vi "SetStyle.vi"(8 "error in (no error)":errorcluster, 10 "Style":T1(ring), 11 "Pen in":refnum<class "Pen.lvclass">) -> (0 "error out":errorcluster, 3 "Pen out":refnum<class "Pen.lvclass">)   [LabVIEW 2021, in "Picture2D.lvlib" / "Pen.lvclass"]
uses:
  Pen.lvclass
  Pen.lvclass/Pen.ctl
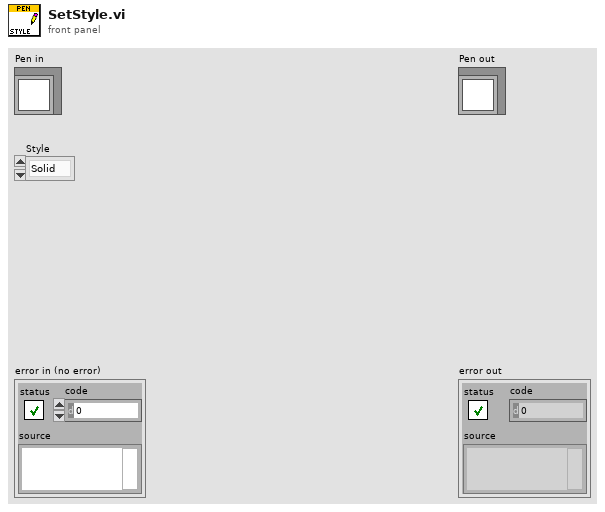
[diagram p1: front panel]
types:
  T1 = enum32{"Solid", "Dash", "Dot", "DashDot", "DashDotDot"}
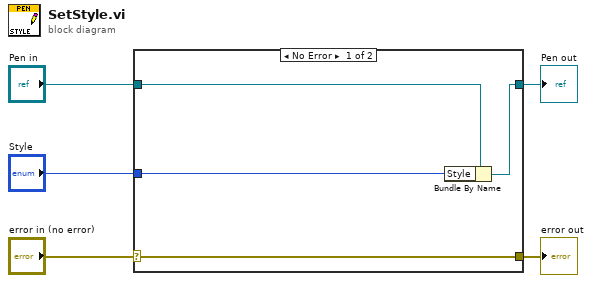
[diagram p0: block diagram]
diagram:
  n1 = case shown="No Error" "error in (no error)" {
    selector: "error in (no error)" -> [w9 w10]
    tunnel: [w9 w10] -> w4
    tunnel: [w7 w11] -> w2
    tunnel: "Pen in" -> [w8 w11]
    tunnel: "Style" -> [w6 _]
    frame No Error {
      n2 = Bundle By Name(cluster=w8, "Style"=w6) -> (w7:refnum<class "Pen.lvclass">)
    }
    frame Error {
    }
  }
  "error out" <- w4
  "Pen out" <- w2
